vi "stepper graphics controller -- V2.vi"(6 "stepper motor state":T2, 7 "slider setter action":T3, 8 "state in":T1, 10 "value":dbl=1.0 format="%#_13g") -> (0 "state OUT":T1)   [LabVIEW 2018]
uses:
  slider setter action.ctl
  stepper motor state.ctl
  slider setter interal state.ctl
  2Dwindow.ctl
  stack action -- control.ctl
  slider action.ctl
  cursor action.ctl
  generate linear region.vi
  generate linear region --complex -- win cen.vi
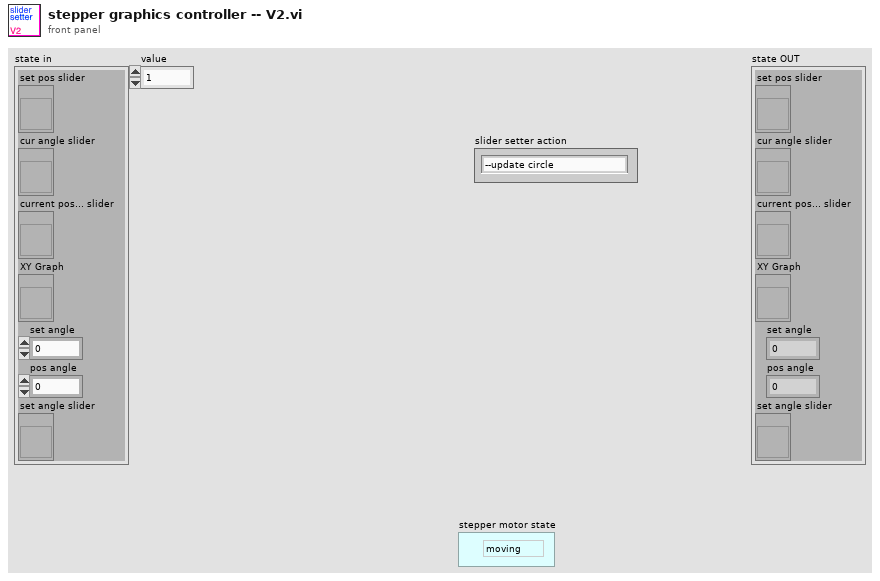
[diagram p1: front panel]
types:
  T1 = typedef "slider setter interal state.ctl" = cluster{"set pos slider":refnum<vi>, "cur angle slider":refnum<vi>, "current pos... slider":refnum<vi>, "XY Graph":refnum<vi>, "set angle":dbl, "pos angle":dbl, "set angle slider":refnum<vi>}
  T2 = typedef "stepper motor state.ctl" = enum16{"moving", "stopped"}
  T3 = typedef "slider setter action.ctl" = enum16{"--update circle", "set step slider moves", "cursor moves", "current pos changed", "init", "void", "--draw current lie", "--draw set line", "--move current step slider", "--move set step slider", "--draw limit lines", "check", "--move set angle slider", "--move current angle slider", "set angle slider moves", "--move cursor", "set set step", "set current step"}
  T4 = typedef "stack action -- control.ctl" = enum16{"push", "pop", "check", "init"}
  T5 = typedef "2Dwindow.ctl" = cluster{"window y":dbl, "center x":dbl, "center y":dbl, "window x":dbl}
  T6 = typedef "slider action.ctl" = enum16{"check", "copy range", "set from value", "set from ratio", "set from slider", "read using other slider"}
  T7 = typedef "cursor action.ctl" = enum16{"range", "read", "write", "check", "zoom out", "smart zoom out", "zoom to aspect ratio 1", "zoom to win", "zoom out 20%", "zoom in 20%", "-empty", "smart zoom out&aspect", "move range left 20%", "move range right 20%", "move range up 20%", "move range down 20%", "zoom to X win", "zoom to Y win", "zoom out X", "zoom out Y", "zoom in X", "zoom in Y", "check plot scale"}
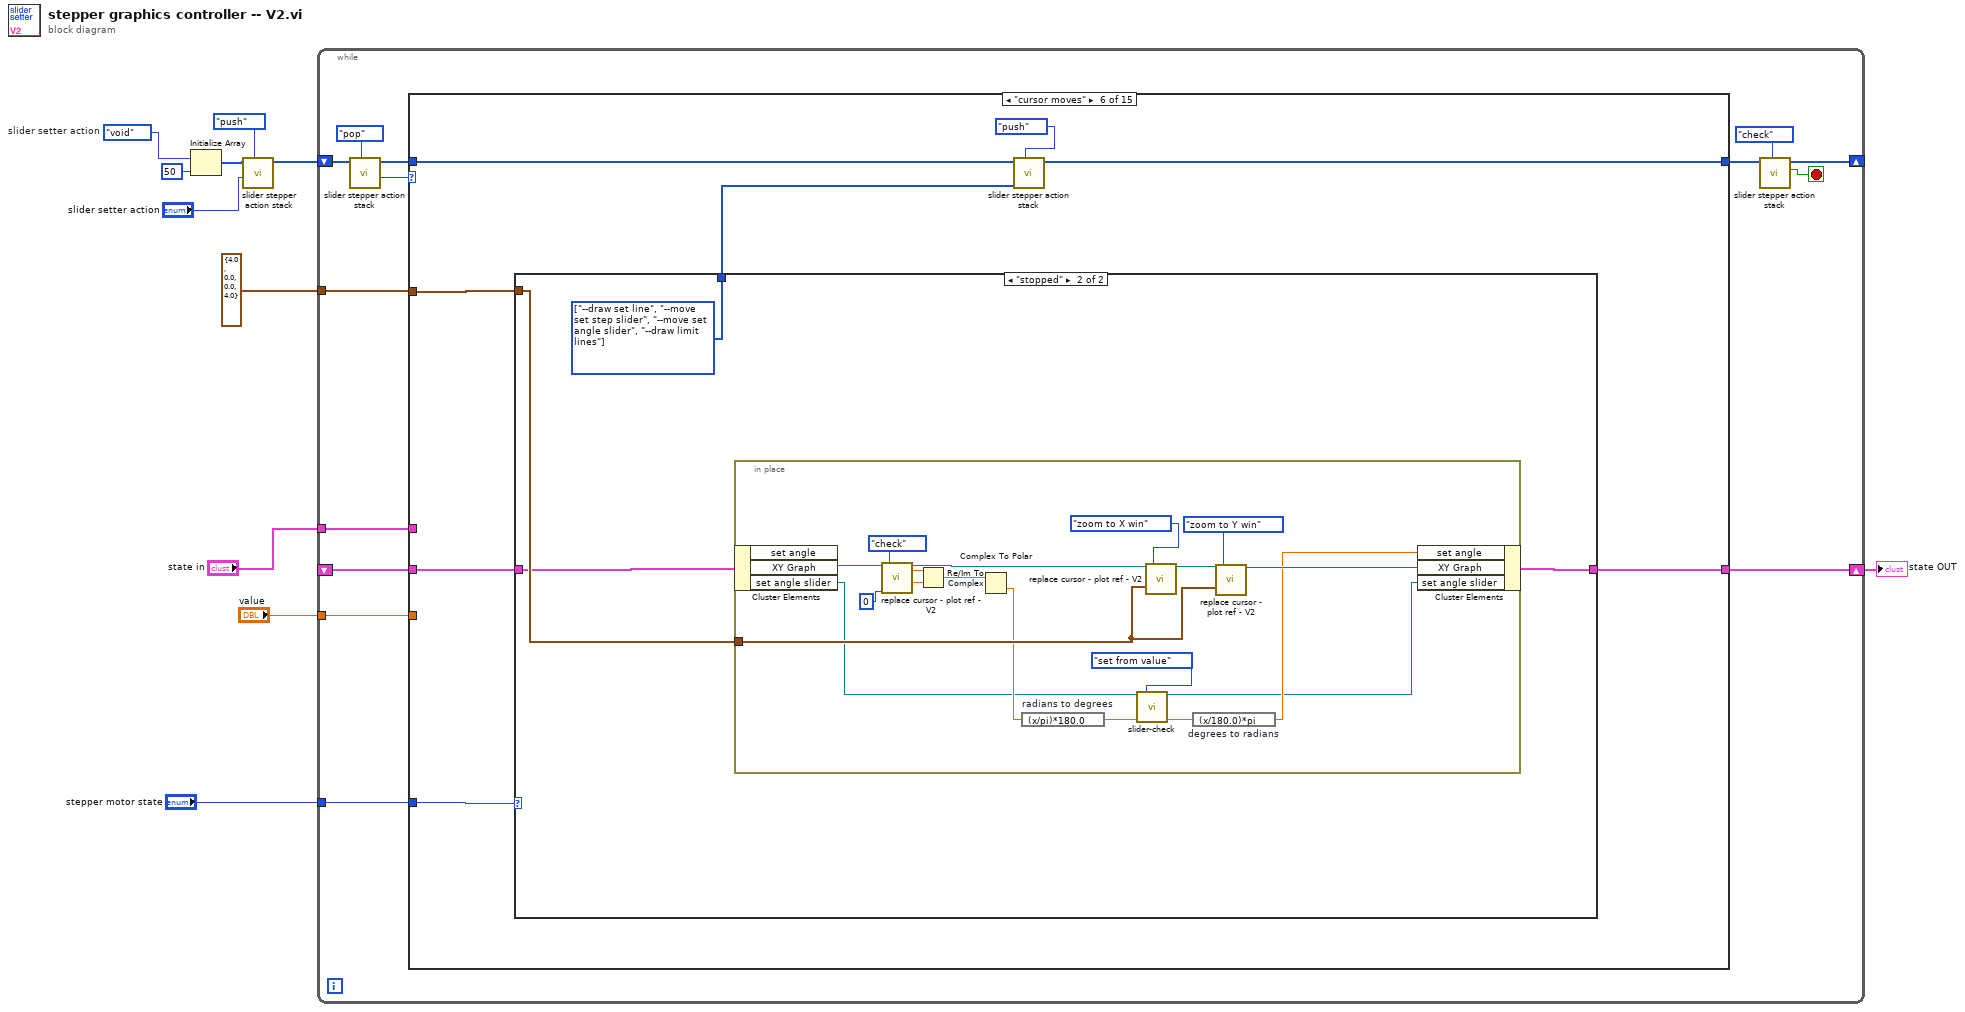
[diagram p0: block diagram]
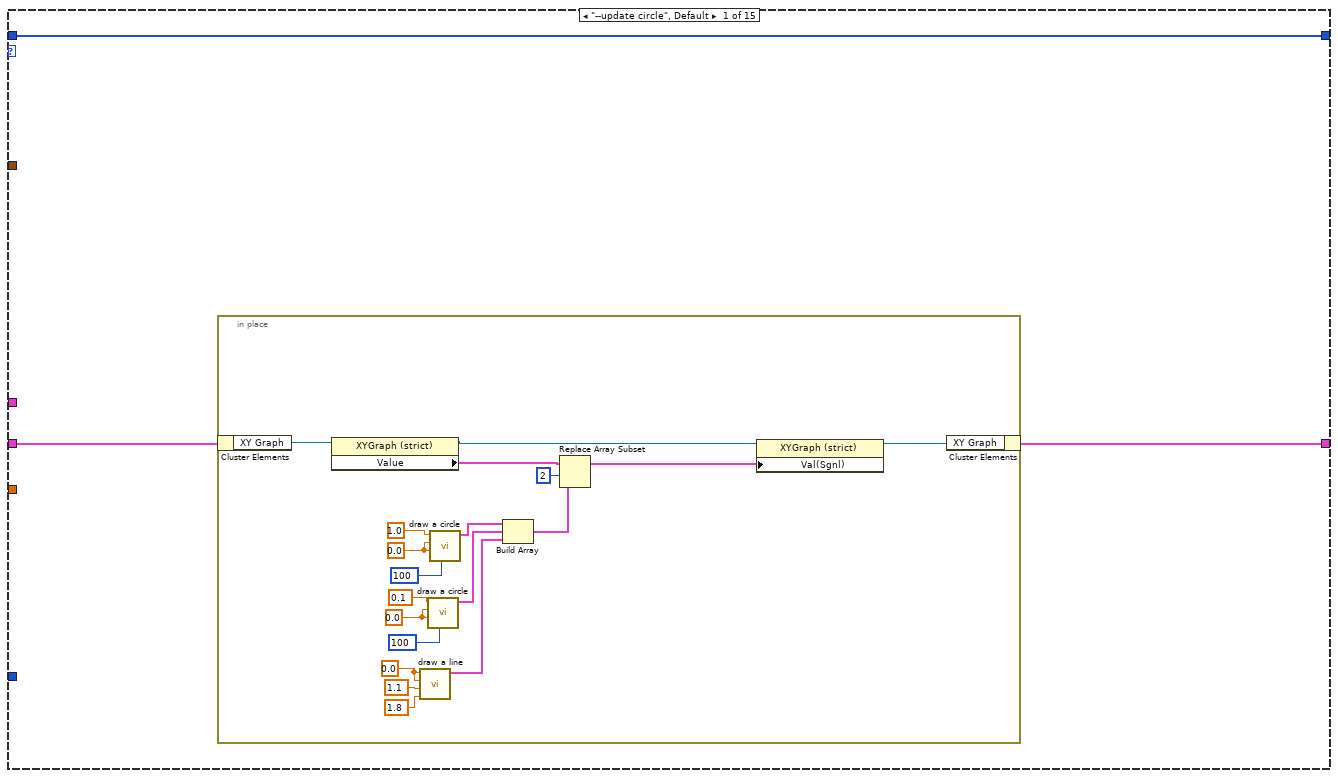
[diagram p2: hidden frame]
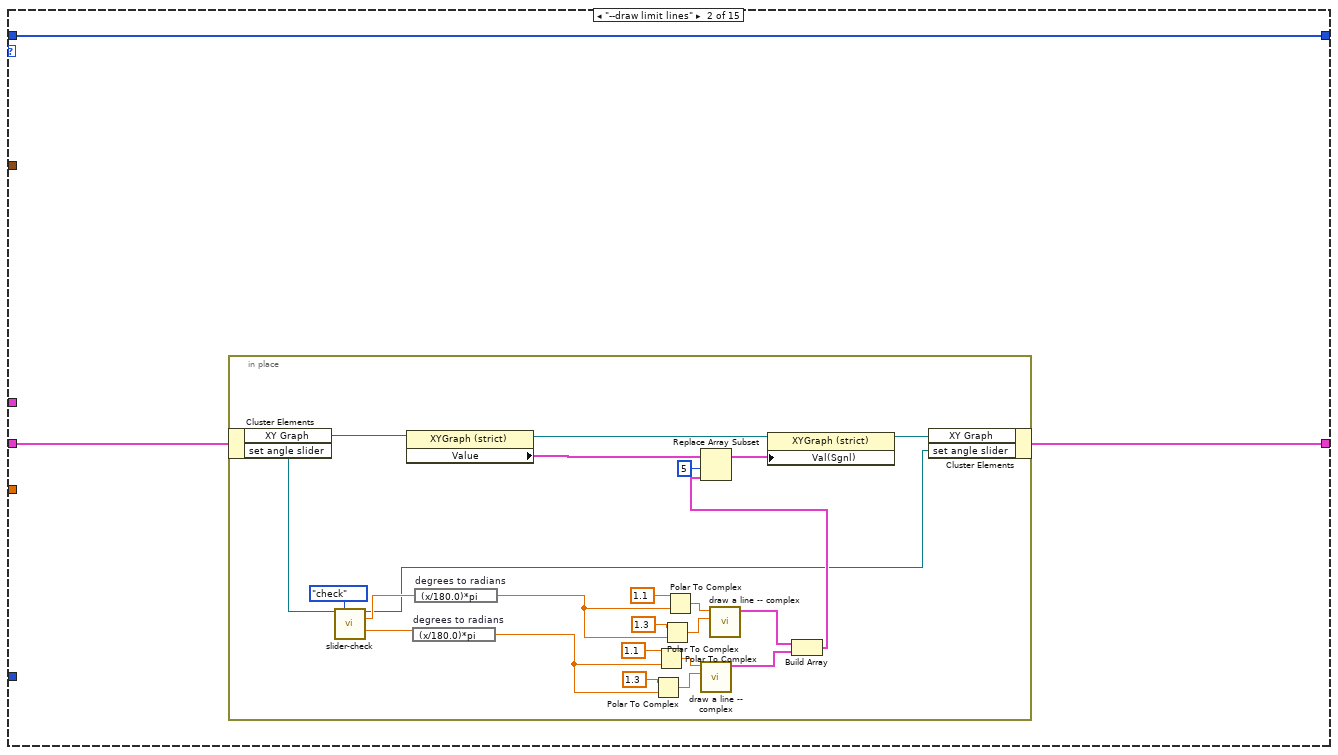
[diagram p3: hidden frame]
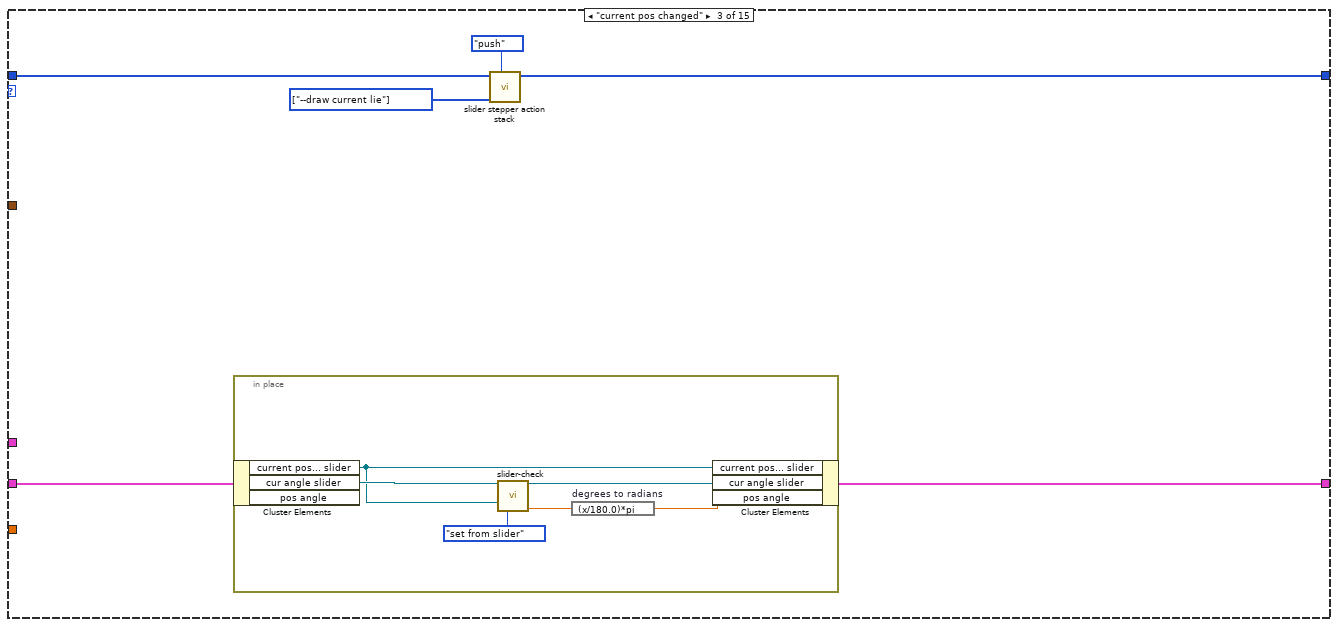
[diagram p4: hidden frame]
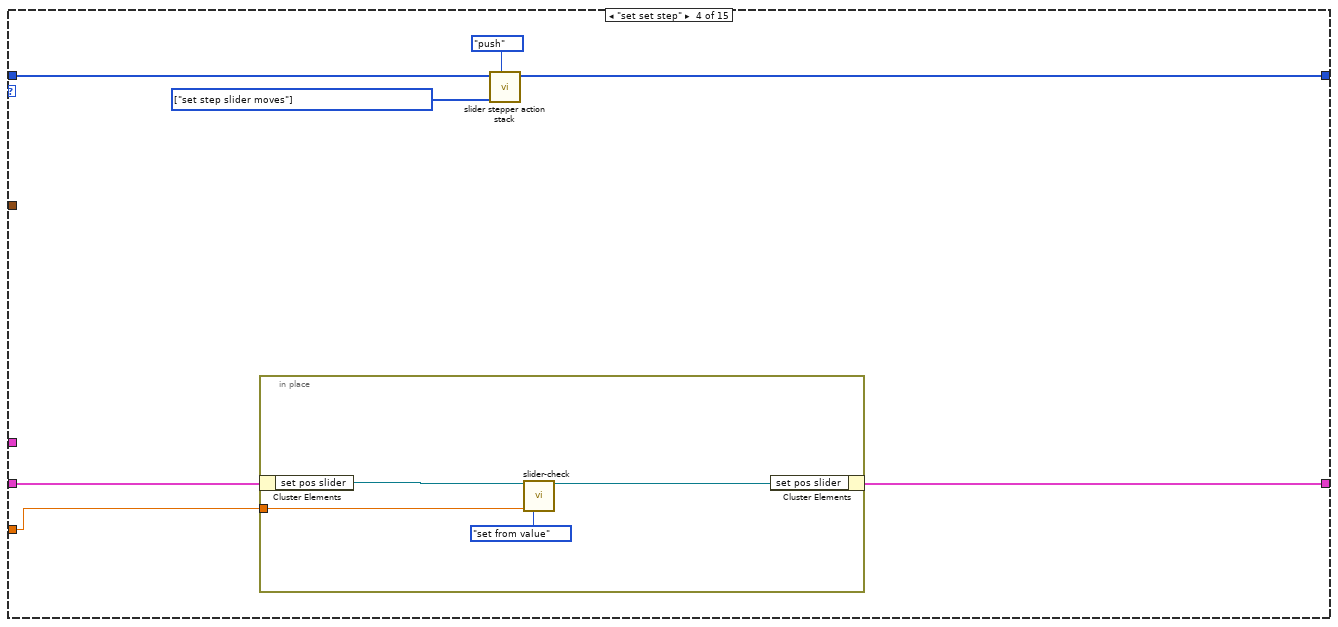
[diagram p5: hidden frame]
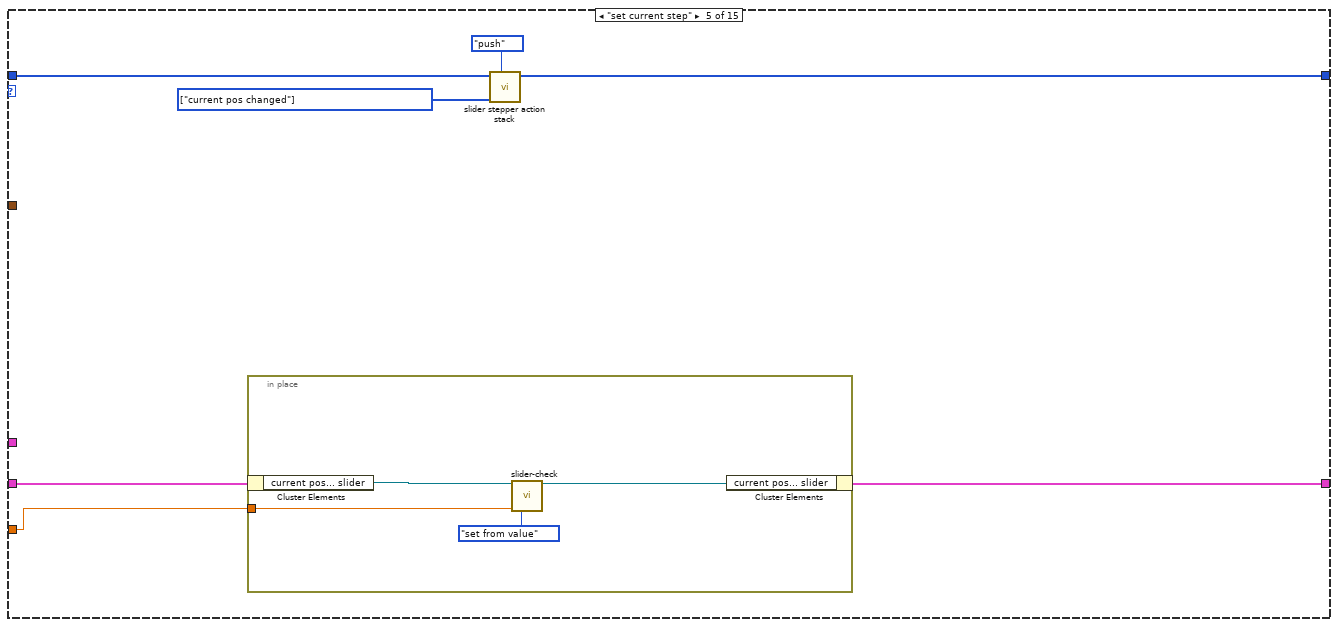
[diagram p6: hidden frame]
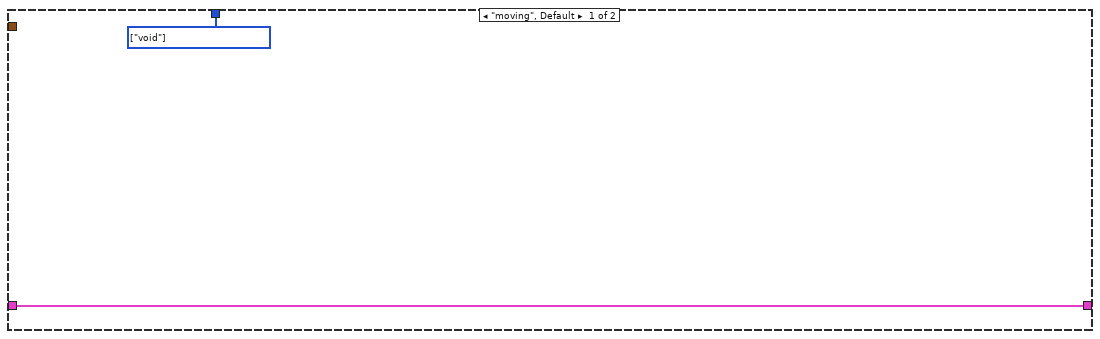
[diagram p7: hidden frame]
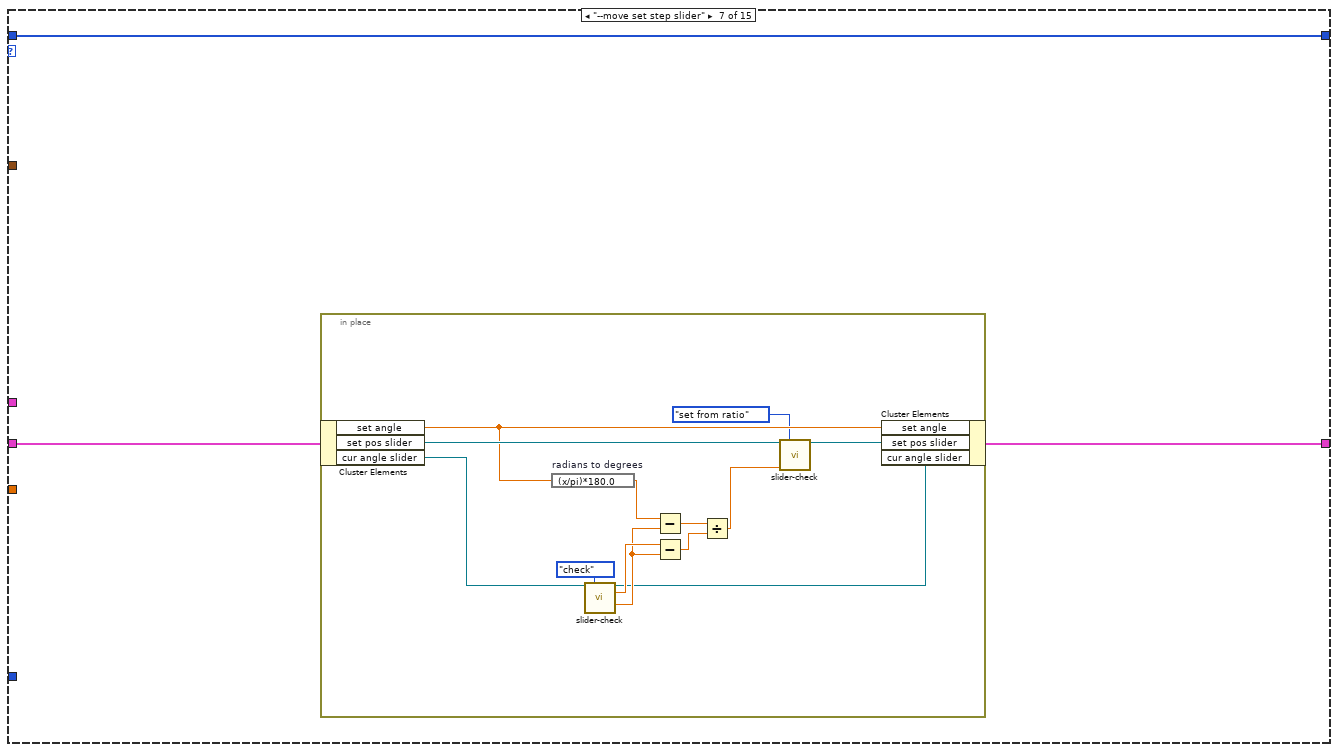
[diagram p8: hidden frame]
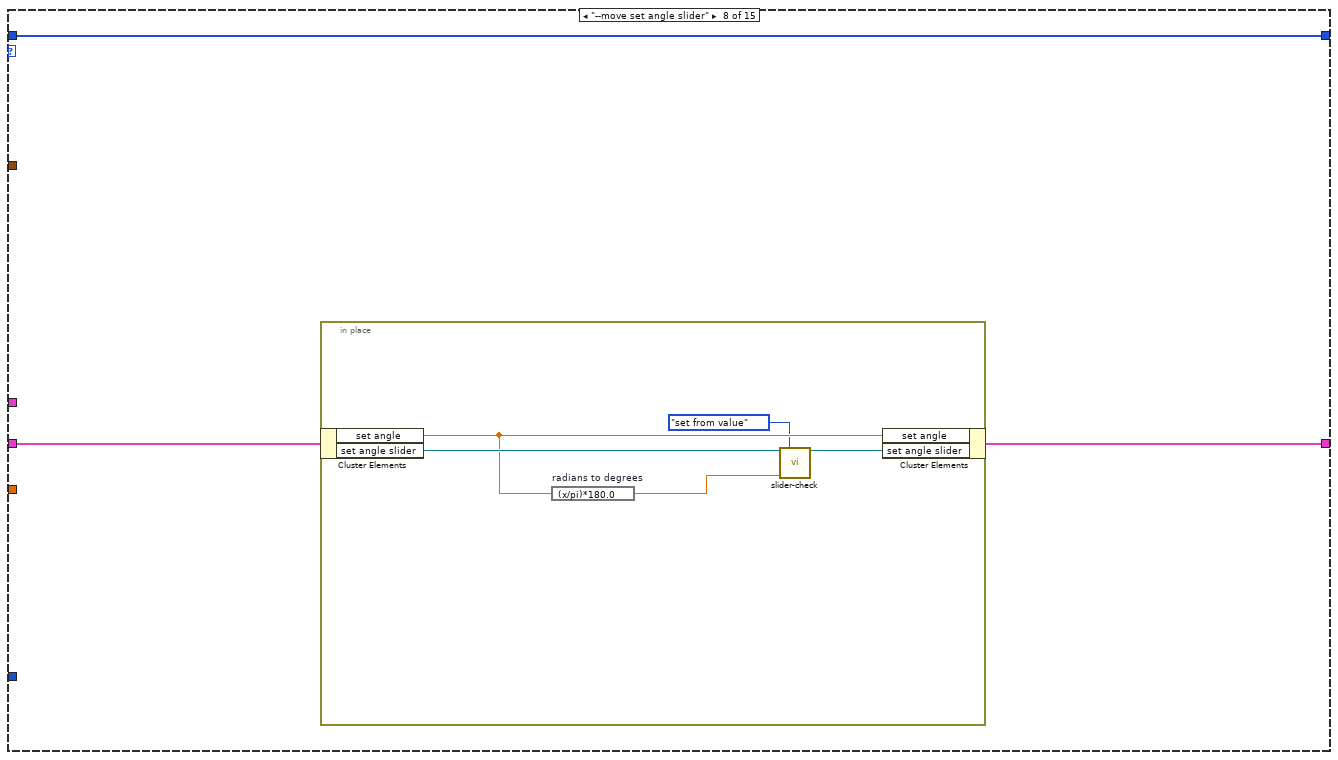
[diagram p9: hidden frame]
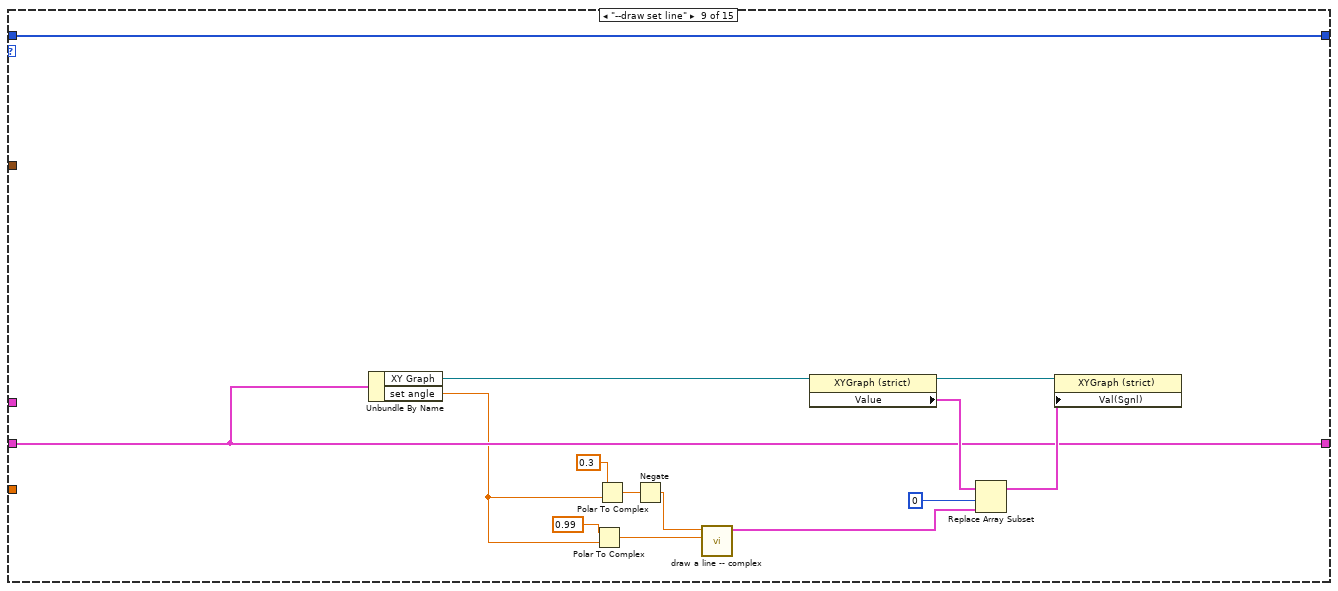
[diagram p10: hidden frame]
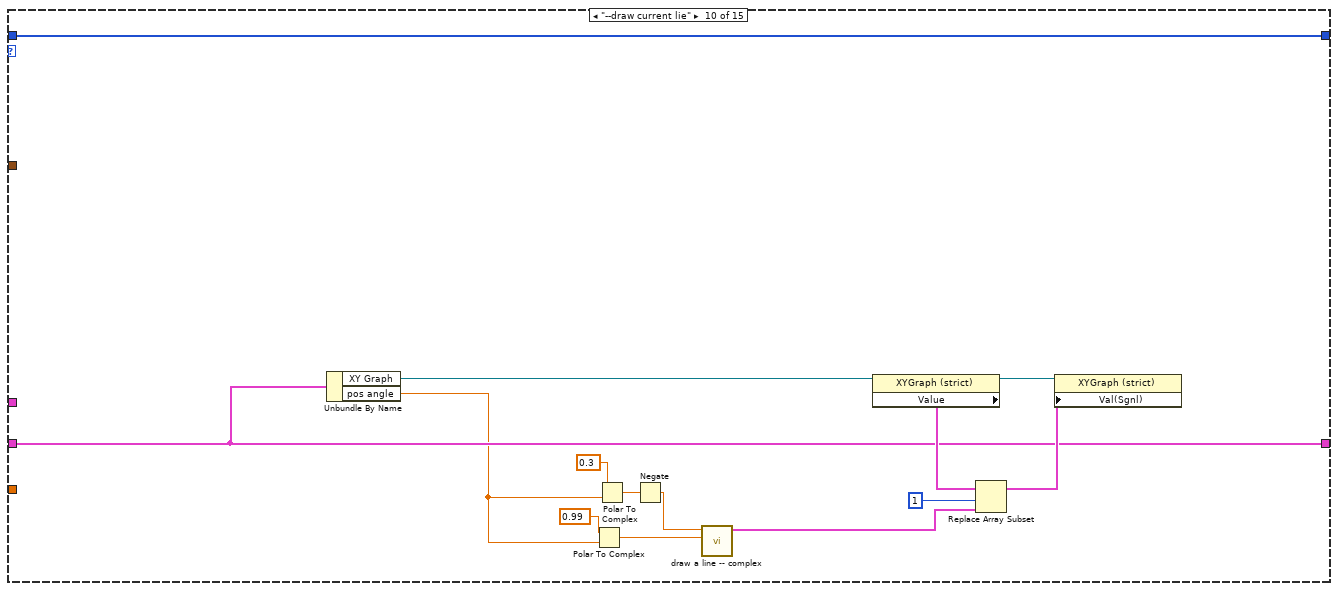
[diagram p11: hidden frame]
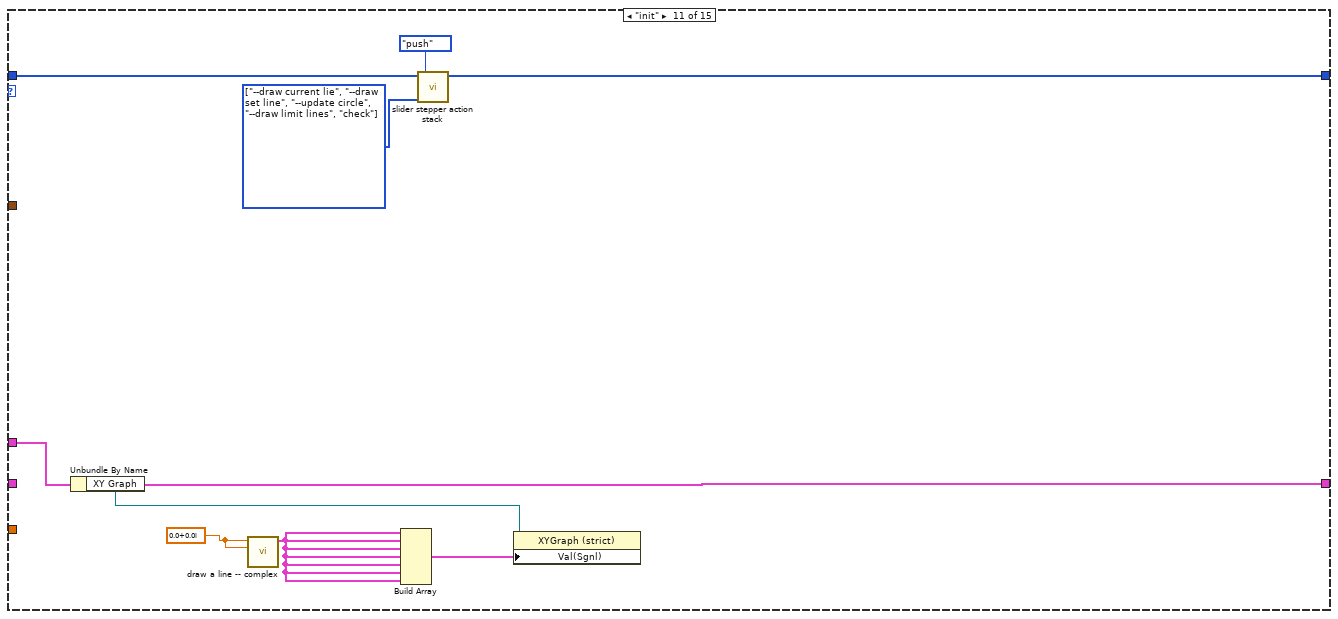
[diagram p12: hidden frame]
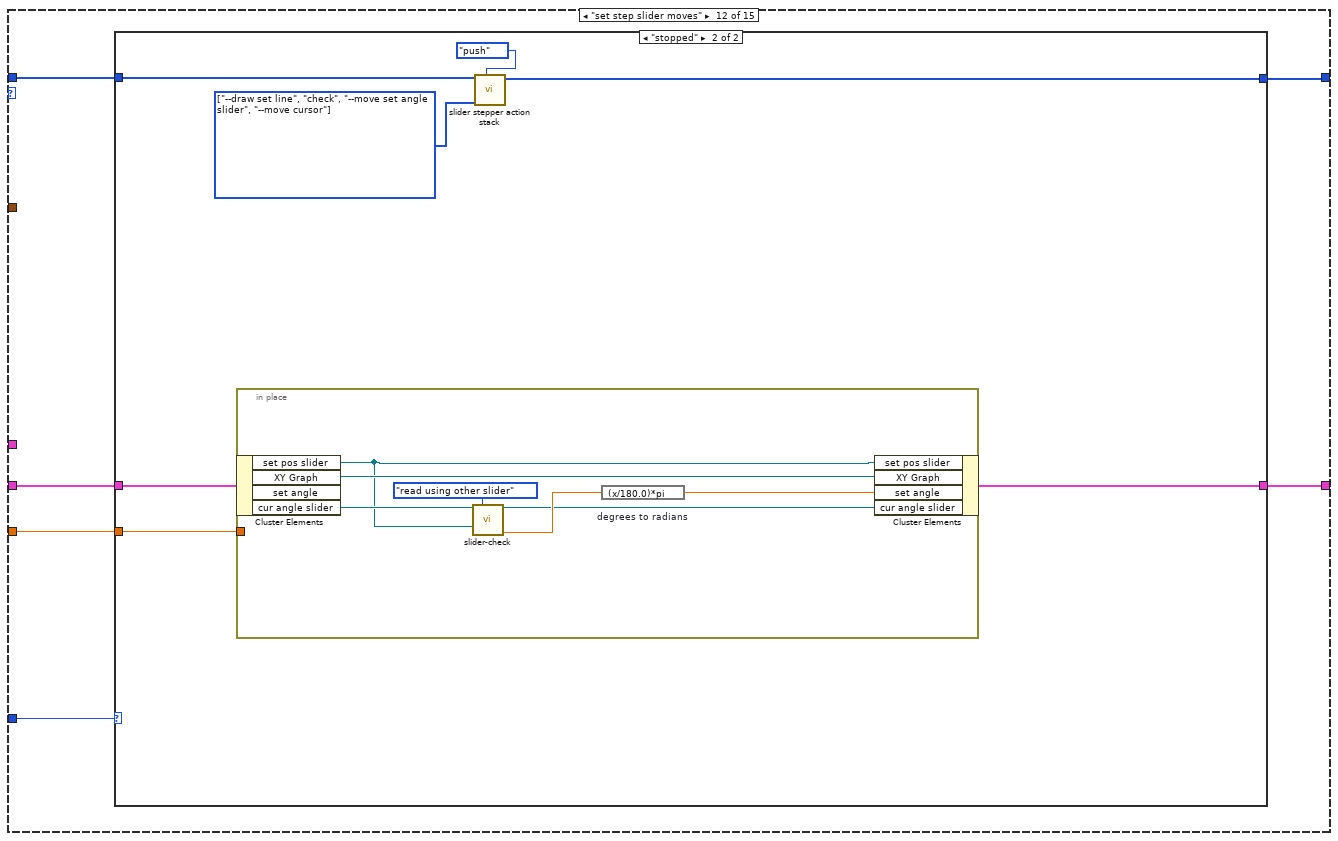
[diagram p13: hidden frame]
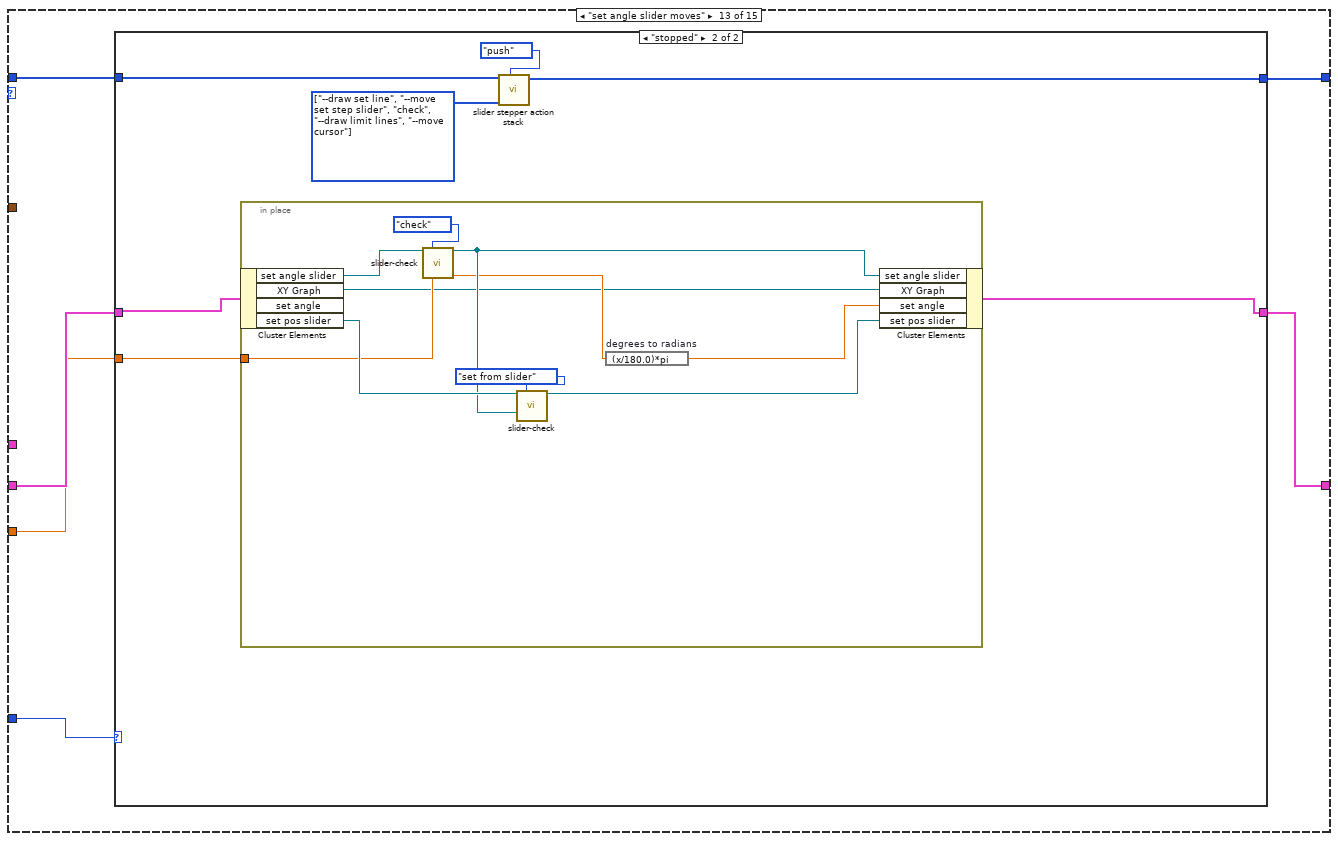
[diagram p15: hidden frame]
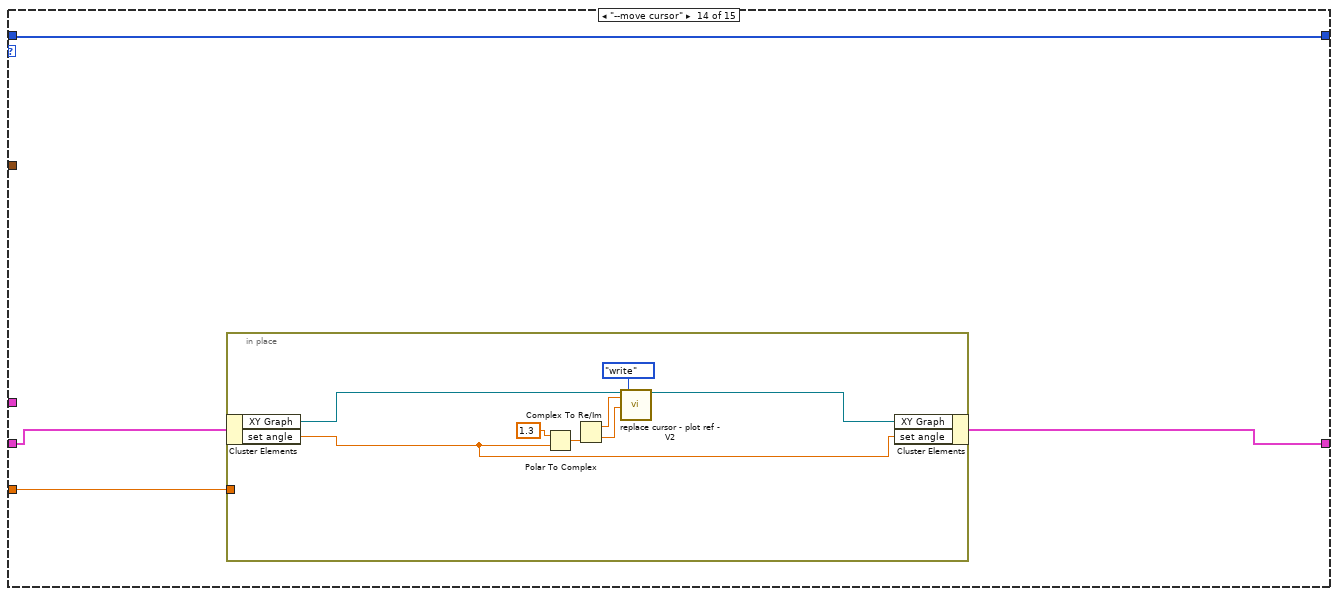
[diagram p17: hidden frame]
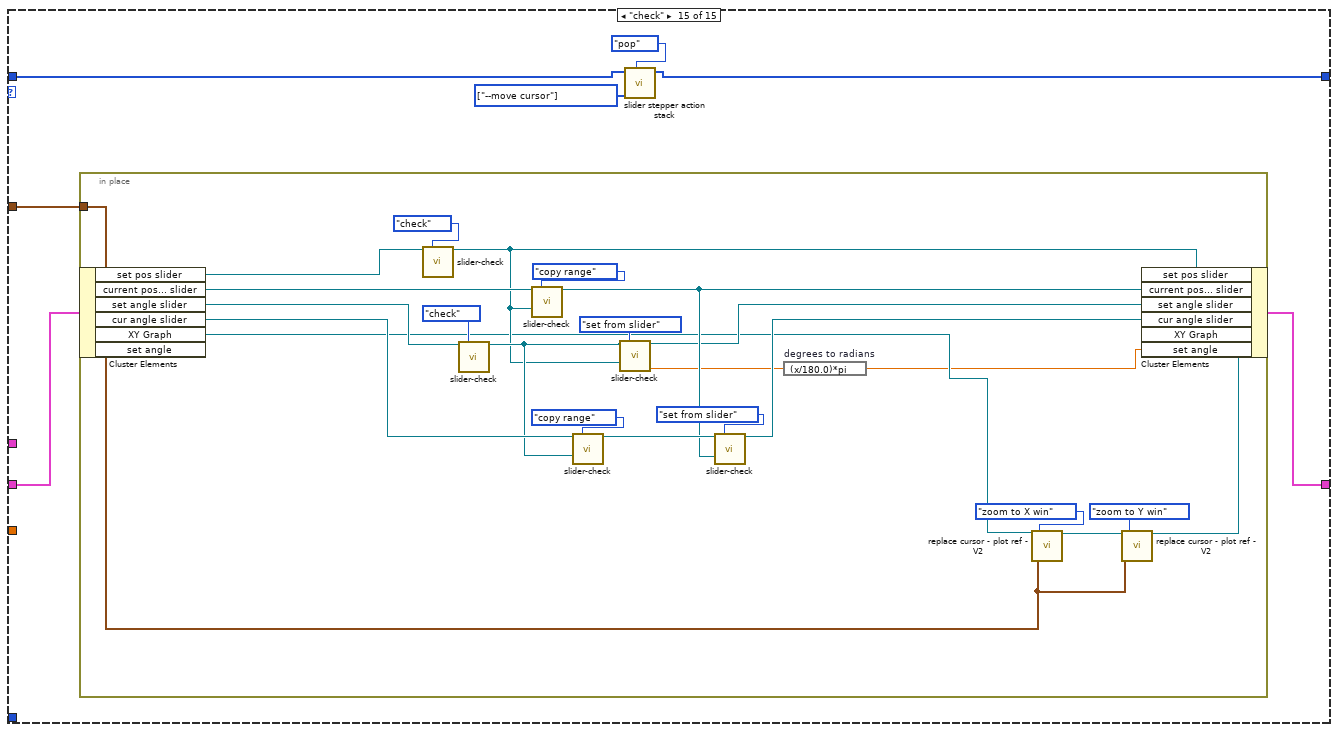
[diagram p18: hidden frame]
diagram:
  w8 = slider_setter_action."void"  # slider setter action
  n1 = Initialize Array(w8, 50 ("dimension size")) -> (w7:T3[])
  n2 = call "slider stepper action stack.vi"("stack action"=stack_action_--_control."push", "slider setter action"="slider setter action", "command stack In"=w7) -> ("command stack OUT"=w5:T3[])  [unwired: 6 in, 2 out]
  n3 = while {
    tunnel: "stepper motor state" -> [w25]
    tunnel: T5 {"window y"=4.0, "center x"=0.0, "center y"=0.0, "window x"=4.0} ("window IN") -> [w24]
    shift-right: [w18] -> _
    shift-left: w5 -> [w22]
    tunnel: "state in" -> [w15]
    shift-right: [w14] -> w2
    shift-left: _ -> [w13]
    tunnel: "value" -> [w12]
    stop <- w16 stop-if-true
    n4 = call "slider stepper action stack.vi"("stack action"=stack_action_--_control."pop", "command stack In"=w22) -> ("slider setter action OUT"=w20:T3, "command stack OUT"=w21:T3[])  [unwired: 7 in, 1 out]
    n5 = case shown="\"cursor moves\"" w20 {
      tunnel: w25 -> [_ _ _ _ _ w116 _ _ _ _ _ w208 w230 _ _]
      tunnel: w24 -> [_ _ _ _ _ w115 _ _ _ _ _ _ _ _ w266]
      tunnel: w21 -> [w28 w50 w80 w93 w104 w113 w142 w158 w179 w193 w201 w207 w229 w250 w265]
      tunnel: [w28 w50 w79 w92 w103 w112 w142 w158 w179 w193 w200 w206 w228 w250 w264] -> w19
      tunnel: w15 -> [_ _ _ _ _ _ _ _ _ _ w195 _ _ _ _]
      tunnel: [w26 w48 w75 w88 w99 w111 w143 w159 w168 w182 w195 w205 w227 w253 w268] -> w14
      tunnel: w13 -> [w27 w49 w76 w89 w100 w110 w144 w160 w168 w182 _ w204 w226 w252 w267]
      tunnel: w12 -> [_ _ _ w87 w98 _ _ _ _ _ _ w203 w225 w251 _]
      frame "--update circle", Default {
        n6 = in-place {
          w41 = 0.0 ("center x")
          w44 = 0.0 ("x0")
          w47 = 0.0 ("center x")
          n7 = in-place-cluster #1(w27) -> ("XY Graph"=w37:refnum<vi>)
          n8 = property class="XYGraph (strict)"(reference=w37) -> (reference out=w36:refnum<vi>, "Value"=w35:cluster{dbl[], dbl[]}[])  [unwired: 1 in, 1 out]
          n9 = call "draw a line.vi"("y1"=1.8 ("x0"), "y0"=1.1 ("x0"), "x1"=w44, "x0"=w44) -> ("output cluster"=w31:cluster{dbl[], dbl[]})  [unwired: 7 in]
          n10 = call "draw a circle.vi"("number of points"=100, "center Y"=w41, "center x"=w41, "radius"=0.1) -> ("output cluster"=w32:cluster{dbl[], dbl[]})  [unwired: 7 in]
          n11 = call "draw a circle.vi"("number of points"=100, "center Y"=w47, "center x"=w47, "radius"=1.0) -> ("output cluster"=w33:cluster{dbl[], dbl[]})  [unwired: 7 in]
          n12 = Build Array(w33, w32, w31) -> (w30:cluster{dbl[], dbl[]}[])
          n13 = Replace Array Subset(array=w35, new element=w30, index=2) -> (w29:cluster{dbl[], dbl[]}[])
          n14 = property class="XYGraph (strict)"(reference=w36, "Val(Sgnl)"=w29) -> (reference out=w38:refnum<vi>)  [unwired: 1 in, 1 out]
          n15 = in-place-cluster #1("XY Graph"=w38) -> (w26:T1)
        }
      }
      frame "--draw limit lines" {
        n16 = in-place {
          n17 = in-place-cluster #2(w49) -> ("XY Graph"=w73:refnum<vi>, "set angle slider"=w67:refnum<vi>)
          n18 = call "slider-check.vi"("slider"=w67, "slider action"=slider_action."check") -> ("slider OUT"=w51:refnum<vi>, "max"=w66:dbl, "min"=w65:dbl)  [unwired: 9 in, 2 out]
          n19 = property class="XYGraph (strict)"(reference=w73) -> (reference out=w72:refnum<vi>, "Value"=w71:cluster{dbl[], dbl[]}[])  [unwired: 1 in, 1 out]
          n20 = expression code="(x/180.0)*pi" "degrees to radians"(w65) -> (w55:dbl)
          n21 = expression code="(x/180.0)*pi" "degrees to radians"(w66) -> (w61:dbl)
          n22 = Polar To Complex(1:w55, 2:1.3 ("x")) -> (0:w57:cdb)
          n23 = Polar To Complex(1:w55, 2:1.1 ("x")) -> (0:w56:cdb)
          n24 = Polar To Complex(1:w61, 2:1.3 ("x")) -> (0:w62:cdb)
          n25 = Polar To Complex(1:w61, 2:1.1 ("x")) -> (0:w60:cdb)
          n26 = call "draw a line -- complex.vi"("x1"=w57, "x0"=w56) -> ("output cluster"=w53:cluster{dbl[], dbl[]})  [unwired: 9 in]
          n27 = call "draw a line -- complex.vi"("x1"=w62, "x0"=w60) -> ("output cluster"=w54:cluster{dbl[], dbl[]})  [unwired: 9 in]
          n28 = Build Array(w54, w53) -> (w52:cluster{dbl[], dbl[]}[])
          n29 = Replace Array Subset(array=w71, new element=w52, index=5) -> (w69:cluster{dbl[], dbl[]}[])
          n30 = property class="XYGraph (strict)"(reference=w72, "Val(Sgnl)"=w69) -> (reference out=w74:refnum<vi>)  [unwired: 1 in, 1 out]
          n31 = in-place-cluster #2("XY Graph"=w74, "set angle slider"=w51) -> (w48:T1)
        }
      }
      frame "current pos changed" {
        w77 = T3[] [enum."--draw current lie"] items=["--update circle", "set step slider moves", "cursor moves", "current pos changed", "init", "void", "--draw current lie", "--draw set line", "--move current step slider", "--move set step slider", "--draw limit lines", "check", "--move set angle slider", "--move current angle slider", "set angle slider moves", "--move cursor", "set set step", "set current step"] ("action list IN")
        n32 = in-place {
          n33 = in-place-cluster #3(w76) -> ("current pos... slider"=w81:refnum<vi>, "cur angle slider"=w86:refnum<vi>)  [unwired: 1 out]
          n34 = call "slider-check.vi"("slider"=w86, "slider action"=slider_action."set from slider", "slider from"=w81) -> ("slider OUT"=w83:refnum<vi>, "value OUT"=w85:dbl)  [unwired: 8 in, 3 out]
          n35 = expression code="(x/180.0)*pi" "degrees to radians"(w85) -> (w84:dbl)
          n36 = in-place-cluster #3("current pos... slider"=w81, "cur angle slider"=w83, "pos angle"=w84) -> (w75:T1)
        }
        n37 = call "slider stepper action stack.vi"("stack action"=stack_action_--_control."push", "action list IN"=w77, "command stack In"=w80) -> ("command stack OUT"=w79:T3[])  [unwired: 6 in, 2 out]
      }
      frame "set set step" {
        w90 = T3[] [enum."set step slider moves"] items=["--update circle", "set step slider moves", "cursor moves", "current pos changed", "init", "void", "--draw current lie", "--draw set line", "--move current step slider", "--move set step slider", "--draw limit lines", "check", "--move set angle slider", "--move current angle slider", "set angle slider moves", "--move cursor", "set set step", "set current step"] ("action list IN")
        n38 = in-place {
          in-place-border: w87 -> [w94]
          n39 = in-place-cluster #4(w89) -> ("set pos slider"=w97:refnum<vi>)
          n40 = call "slider-check.vi"("slider"=w97, "slider action"=slider_action."set from value", "value IN"=w94) -> ("slider OUT"=w96:refnum<vi>)  [unwired: 8 in, 4 out]
          n41 = in-place-cluster #4("set pos slider"=w96) -> (w88:T1)
        }
        n42 = call "slider stepper action stack.vi"("stack action"=stack_action_--_control."push", "action list IN"=w90, "command stack In"=w93) -> ("command stack OUT"=w92:T3[])  [unwired: 6 in, 2 out]
      }
      frame "set current step" {
        w101 = T3[] [enum."current pos changed"] items=["--update circle", "set step slider moves", "cursor moves", "current pos changed", "init", "void", "--draw current lie", "--draw set line", "--move current step slider", "--move set step slider", "--draw limit lines", "check", "--move set angle slider", "--move current angle slider", "set angle slider moves", "--move cursor", "set set step", "set current step"] ("action list IN")
        n43 = in-place {
          in-place-border: w98 -> [w105]
          n44 = in-place-cluster #5(w100) -> ("current pos... slider"=w108:refnum<vi>)
          n45 = call "slider-check.vi"("slider"=w108, "slider action"=slider_action."set from value", "value IN"=w105) -> ("slider OUT"=w107:refnum<vi>)  [unwired: 8 in, 4 out]
          n46 = in-place-cluster #5("current pos... slider"=w107) -> (w99:T1)
        }
        n47 = call "slider stepper action stack.vi"("stack action"=stack_action_--_control."push", "action list IN"=w101, "command stack In"=w104) -> ("command stack OUT"=w103:T3[])  [unwired: 6 in, 2 out]
      }
      frame "cursor moves" {
        n48 = case shown="\"stopped\"" w116 {
          tunnel: w115 -> [_ w122]
          tunnel: [w118 w121] -> w111
          tunnel: w110 -> [w118 w120]
          tunnel: [w117 w119] -> w109
          frame "moving", Default {
            w117 = T3[] [enum."void"] items=["--update circle", "set step slider moves", "cursor moves", "current pos changed", "init", "void", "--draw current lie", "--draw set line", "--move current step slider", "--move set step slider", "--draw limit lines", "check", "--move set angle slider", "--move current angle slider", "set angle slider moves", "--move cursor", "set set step", "set current step"] ("action list IN")
          }
          frame "stopped" {
            w119 = T3[] [enum."--draw set line", enum."--move set step slider", enum."--move set angle slider", enum."--draw limit lines"] items=["--update circle", "set step slider moves", "cursor moves", "current pos changed", "init", "void", "--draw current lie", "--draw set line", "--move current step slider", "--move set step slider", "--draw limit lines", "check", "--move set angle slider", "--move current angle slider", "set angle slider moves", "--move cursor", "set set step", "set current step"] ("action list IN")
            n49 = in-place {
              in-place-border: w122 -> [w134]
              n50 = in-place-cluster #6(w120) -> ("XY Graph"=w132:refnum<vi>, "set angle slider"=w128:refnum<vi>)  [unwired: 1 out]
              n51 = call "replace cursor - plot ref - V2.vi"("Plot ref in"=w132, "cursor index"=0, "cursor action"=cursor_action."check") -> ("Plot ref out"=w133:refnum<vi>, "read X"=w139:dbl, "read Y"=w138:dbl)  [unwired: 13 in, 1 out]
              n52 = Re/Im To Complex(1:w138, 2:w139) -> (0:w137:cdb)
              n53 = Complex To Polar(r * e^(i*theta)=w137) -> (theta=w129:dbl)  [unwired: 1 out]
              n54 = expression code="(x/pi)*180.0" "radians to degrees"(w129) -> (w127:dbl)
              n55 = call "slider-check.vi"("slider"=w128, "slider action"=slider_action."set from value", "value IN"=w127) -> ("slider OUT"=w123:refnum<vi>, "value OUT"=w125:dbl)  [unwired: 8 in, 3 out]
              n56 = call "replace cursor - plot ref - V2.vi"("Plot ref in"=w133, "window IN"=w134, "cursor action"=cursor_action."zoom to X win") -> ("Plot ref out"=w131:refnum<vi>)  [unwired: 13 in, 3 out]
              n57 = expression code="(x/180.0)*pi" "degrees to radians"(w125) -> (w124:dbl)
              n58 = call "replace cursor - plot ref - V2.vi"("Plot ref in"=w131, "window IN"=w134, "cursor action"=cursor_action."zoom to Y win") -> ("Plot ref out"=w130:refnum<vi>)  [unwired: 13 in, 3 out]
              n59 = in-place-cluster #6("set angle"=w124, "XY Graph"=w130, "set angle slider"=w123) -> (w121:T1)
            }
          }
        }
        n60 = call "slider stepper action stack.vi"("stack action"=stack_action_--_control."push", "action list IN"=w109, "command stack In"=w113) -> ("command stack OUT"=w112:T3[])  [unwired: 6 in, 2 out]
      }
      frame "--move set step slider" {
        n61 = in-place {
          n62 = in-place-cluster #7(w144) -> ("set angle"=w147:dbl, "set pos slider"=w149:refnum<vi>, "cur angle slider"=w150:refnum<vi>)
          n63 = expression code="(x/pi)*180.0" "radians to degrees"(w147) -> (w151:dbl)
          n64 = call "slider-check.vi"("slider"=w150, "slider action"=slider_action."check") -> ("slider OUT"=w146:refnum<vi>, "max"=w156:dbl, "min"=w155:dbl)  [unwired: 9 in, 2 out]
          n65 = Subtract(x=w151, y=w155) -> (x-y=w154:dbl)
          n66 = Subtract(x=w156, y=w155) -> (x-y=w153:dbl)
          n67 = Divide(x=w154, y=w153) -> (x/y=w152:dbl)
          n68 = call "slider-check.vi"("slider"=w149, "slider action"=slider_action."set from ratio", "value IN"=w152) -> ("slider OUT"=w148:refnum<vi>)  [unwired: 8 in, 4 out]
          n69 = in-place-cluster #7("set angle"=w147, "set pos slider"=w148, "cur angle slider"=w146) -> (w143:T1)
        }
      }
      frame "--move set angle slider" {
        n70 = in-place {
          n71 = in-place-cluster #8(w160) -> ("set angle"=w163:dbl, "set angle slider"=w165:refnum<vi>)
          n72 = expression code="(x/pi)*180.0" "radians to degrees"(w163) -> (w162:dbl)
          n73 = call "slider-check.vi"("slider"=w165, "slider action"=slider_action."set from value", "value IN"=w162) -> ("slider OUT"=w164:refnum<vi>)  [unwired: 8 in, 4 out]
          n74 = in-place-cluster #8("set angle"=w163, "set angle slider"=w164) -> (w159:T1)
        }
      }
      frame "--draw set line" {
        n75 = Unbundle By Name(w168) -> ("XY Graph"=w166:refnum<vi>, "set angle"=w167:dbl)
        n76 = Polar To Complex(1:w167, 2:0.99 ("x")) -> (0:w170:cdb)
        n77 = Polar To Complex(1:w167, 2:0.3 ("x")) -> (0:w172:cdb)
        n78 = Negate(x=w172) -> (-x=w171:cdb)
        n79 = call "draw a line -- complex.vi"("x1"=w170, "x0"=w171) -> ("output cluster"=w169:cluster{dbl[], dbl[]})  [unwired: 9 in]
        n80 = property class="XYGraph (strict)"(reference=w166) -> (reference out=w178:refnum<vi>, "Value"=w177:cluster{dbl[], dbl[]}[])  [unwired: 1 in, 1 out]
        n81 = Replace Array Subset(array=w177, new element=w169, index=0) -> (w176:cluster{dbl[], dbl[]}[])
        n82 = property class="XYGraph (strict)"(reference=w178, "Val(Sgnl)"=w176) -> ()  [unwired: 1 in, 2 out]
      }
      frame "--draw current lie" {
        n83 = Unbundle By Name(w182) -> ("XY Graph"=w180:refnum<vi>, "pos angle"=w181:dbl)
        n84 = Polar To Complex(1:w181, 2:0.99 ("x")) -> (0:w184:cdb)
        n85 = Polar To Complex(1:w181, 2:0.3 ("x")) -> (0:w186:cdb)
        n86 = Negate(x=w186) -> (-x=w185:cdb)
        n87 = call "draw a line -- complex.vi"("x1"=w184, "x0"=w185) -> ("output cluster"=w183:cluster{dbl[], dbl[]})  [unwired: 9 in]
        n88 = property class="XYGraph (strict)"(reference=w180) -> (reference out=w192:refnum<vi>, "Value"=w191:cluster{dbl[], dbl[]}[])  [unwired: 1 in, 1 out]
        n89 = Replace Array Subset(array=w191, new element=w183, index=1) -> (w190:cluster{dbl[], dbl[]}[])
        n90 = property class="XYGraph (strict)"(reference=w192, "Val(Sgnl)"=w190) -> ()  [unwired: 1 in, 2 out]
      }
      frame "init" {
        w197 = cdb 0.0+0.0i ("x0")
        w198 = T3[] [enum."--draw current lie", enum."--draw set line", enum."--update circle", enum."--draw limit lines", enum."check"] items=["--update circle", "set step slider moves", "cursor moves", "current pos changed", "init", "void", "--draw current lie", "--draw set line", "--move current step slider", "--move set step slider", "--draw limit lines", "check", "--move set angle slider", "--move current angle slider", "set angle slider moves", "--move cursor", "set set step", "set current step"] ("action list IN")
        n91 = Unbundle By Name(w195) -> ("XY Graph"=w194:refnum<vi>)
        n92 = call "draw a line -- complex.vi"("x1"=w197, "x0"=w197) -> ("output cluster"=w196:cluster{dbl[], dbl[]})  [unwired: 9 in]
        n93 = Build Array(w196, w196, w196, w196, w196, w196, w196) -> (w202:cluster{dbl[], dbl[]}[])
        n94 = call "slider stepper action stack.vi"("stack action"=stack_action_--_control."push", "action list IN"=w198, "command stack In"=w201) -> ("command stack OUT"=w200:T3[])  [unwired: 6 in, 2 out]
        n95 = property class="XYGraph (strict)"(reference=w194, "Val(Sgnl)"=w202) -> ()  [unwired: 1 in, 2 out]
      }
      frame "set step slider moves" {
        n96 = case shown="\"stopped\"" w208 {
          tunnel: w207 -> [w210 w217]
          tunnel: [w210 w216] -> w206
          tunnel: w204 -> [w209 w214]
          tunnel: [w209 w213] -> w205
          tunnel: w203 -> [_ w211]
          frame "moving", Default {
          }
          frame "stopped" {
            w215 = T3[] [enum."--draw set line", enum."check", enum."--move set angle slider", enum."--move cursor"] items=["--update circle", "set step slider moves", "cursor moves", "current pos changed", "init", "void", "--draw current lie", "--draw set line", "--move current step slider", "--move set step slider", "--draw limit lines", "check", "--move set angle slider", "--move current angle slider", "set angle slider moves", "--move cursor", "set set step", "set current step"] ("action list IN")
            n97 = in-place {
              in-place-border: w211 -> [_]
              n98 = in-place-cluster #9(w214) -> ("set pos slider"=w220:refnum<vi>, "XY Graph"=w221:refnum<vi>, "cur angle slider"=w223:refnum<vi>)  [unwired: 1 out]
              n99 = call "slider-check.vi"("slider"=w223, "slider action"=slider_action."read using other slider", "slider from"=w220) -> ("slider OUT"=w218:refnum<vi>, "value OUT"=w219:dbl)  [unwired: 8 in, 3 out]
              n100 = expression code="(x/180.0)*pi" "degrees to radians"(w219) -> (w222:dbl)
              n101 = in-place-cluster #9("set pos slider"=w220, "XY Graph"=w221, "set angle"=w222, "cur angle slider"=w218) -> (w213:T1)
            }
            n102 = call "slider stepper action stack.vi"("stack action"=stack_action_--_control."push", "action list IN"=w215, "command stack In"=w217) -> ("command stack OUT"=w216:T3[])  [unwired: 6 in, 2 out]
          }
        }
      }
      frame "set angle slider moves" {
        n103 = case shown="\"stopped\"" w230 {
          tunnel: w229 -> [w232 w239]
          tunnel: [w232 w238] -> w228
          tunnel: w226 -> [w231 w236]
          tunnel: [w231 w235] -> w227
          tunnel: w225 -> [_ w233]
          frame "moving", Default {
          }
          frame "stopped" {
            w237 = T3[] [enum."--draw set line", enum."--move set step slider", enum."check", enum."--draw limit lines", enum."--move cursor"] items=["--update circle", "set step slider moves", "cursor moves", "current pos changed", "init", "void", "--draw current lie", "--draw set line", "--move current step slider", "--move set step slider", "--draw limit lines", "check", "--move set angle slider", "--move current angle slider", "set angle slider moves", "--move cursor", "set set step", "set current step"] ("action list IN")
            n104 = in-place {
              in-place-border: w233 -> [w244]
              n105 = in-place-cluster #10(w236) -> ("set angle slider"=w247:refnum<vi>, "XY Graph"=w240:refnum<vi>, "set pos slider"=w246:refnum<vi>)  [unwired: 1 out]
              n106 = call "slider-check.vi"("slider"=w247, "slider action"=slider_action."check", "default"=w244) -> ("slider OUT"=w243:refnum<vi>, "value OUT"=w241:dbl)  [unwired: 8 in, 3 out]
              n107 = call "slider-check.vi"("slider"=w246, "slider action"=slider_action."set from slider", "slider from"=w243) -> ("slider OUT"=w242:refnum<vi>)  [unwired: 8 in, 4 out]
              n108 = expression code="(x/180.0)*pi" "degrees to radians"(w241) -> (w245:dbl)
              n109 = in-place-cluster #10("set angle slider"=w243, "XY Graph"=w240, "set angle"=w245, "set pos slider"=w242) -> (w235:T1)
            }
            n110 = call "slider stepper action stack.vi"("stack action"=stack_action_--_control."push", "action list IN"=w237, "command stack In"=w239) -> ("command stack OUT"=w238:T3[])  [unwired: 6 in, 2 out]
          }
        }
      }
      frame "--move cursor" {
        n111 = in-place {
          in-place-border: w251 -> [_]
          n112 = in-place-cluster #11(w252) -> ("XY Graph"=w256:refnum<vi>, "set angle"=w254:dbl)
          n113 = Polar To Complex(1:w254, 2:1.3 ("r")) -> (0:w259:cdb)
          n114 = Complex To Re/Im(x + iy=w259) -> (x=w260:dbl, y=w261:dbl)
          n115 = call "replace cursor - plot ref - V2.vi"("Plot ref in"=w256, "new X"=w260, "new  Y"=w261, "cursor action"=cursor_action."write") -> ("Plot ref out"=w255:refnum<vi>)  [unwired: 12 in, 3 out]
          n116 = in-place-cluster #11("XY Graph"=w255, "set angle"=w254) -> (w253:T1)
        }
      }
      frame "check" {
        w262 = T3[] [enum."--move cursor"] items=["--update circle", "set step slider moves", "cursor moves", "current pos changed", "init", "void", "--draw current lie", "--draw set line", "--move current step slider", "--move set step slider", "--draw limit lines", "check", "--move set angle slider", "--move current angle slider", "set angle slider moves", "--move cursor", "set set step", "set current step"] ("action list IN")
        n117 = in-place {
          in-place-border: w266 -> [w273]
          n118 = in-place-cluster #12(w267) -> ("set pos slider"=w290:refnum<vi>, "current pos... slider"=w288:refnum<vi>, "set angle slider"=w287:refnum<vi>, "cur angle slider"=w286:refnum<vi>, "XY Graph"=w270:refnum<vi>)  [unwired: 1 out]
          n119 = call "slider-check.vi"("slider"=w290, "slider action"=slider_action."check") -> ("slider OUT"=w277:refnum<vi>)  [unwired: 9 in, 4 out]
          n120 = call "slider-check.vi"("slider"=w287, "slider action"=slider_action."check") -> ("slider OUT"=w279:refnum<vi>)  [unwired: 9 in, 4 out]
          n121 = call "slider-check.vi"("slider"=w288, "slider action"=slider_action."copy range", "slider from"=w277) -> ("slider OUT"=w281:refnum<vi>)  [unwired: 8 in, 4 out]
          n122 = call "slider-check.vi"("slider"=w286, "slider action"=slider_action."copy range", "slider from"=w279) -> ("slider OUT"=w284:refnum<vi>)  [unwired: 8 in, 4 out]
          n123 = call "slider-check.vi"("slider"=w279, "slider action"=slider_action."set from slider", "slider from"=w277) -> ("slider OUT"=w278:refnum<vi>, "value OUT"=w274:dbl)  [unwired: 8 in, 3 out]
          n124 = call "slider-check.vi"("slider"=w284, "slider action"=slider_action."set from slider", "slider from"=w281) -> ("slider OUT"=w283:refnum<vi>)  [unwired: 8 in, 4 out]
          n125 = expression code="(x/180.0)*pi" "degrees to radians"(w274) -> (w269:dbl)
          n126 = call "replace cursor - plot ref - V2.vi"("Plot ref in"=w270, "window IN"=w273, "cursor action"=cursor_action."zoom to X win") -> ("Plot ref out"=w275:refnum<vi>)  [unwired: 13 in, 3 out]
          n127 = call "replace cursor - plot ref - V2.vi"("Plot ref in"=w275, "window IN"=w273, "cursor action"=cursor_action."zoom to Y win") -> ("Plot ref out"=w272:refnum<vi>)  [unwired: 13 in, 3 out]
          n128 = in-place-cluster #12("set pos slider"=w277, "current pos... slider"=w281, "set angle slider"=w278, "cur angle slider"=w283, "XY Graph"=w272, "set angle"=w269) -> (w268:T1)
        }
        n129 = call "slider stepper action stack.vi"("stack action"=stack_action_--_control."pop", "action list IN"=w262, "command stack In"=w265) -> ("command stack OUT"=w264:T3[])  [unwired: 6 in, 2 out]
      }
    }
    n130 = call "slider stepper action stack.vi"("stack action"=stack_action_--_control."check", "command stack In"=w19) -> ("stack is empty ?"=w16:bool, "command stack OUT"=w18:T3[])  [unwired: 7 in, 1 out]
  }
  "state OUT" <- w2
